vi "Facade.vi"(0 "Data In":T5 caption="数据输入", 2 "Display State In":T2 caption="显示状态输入", 3 "Container State":T4 caption="容器状态") -> (6 "Data Out":T5 caption="数据输出", 7 "Display State Out":T2 caption="显示状态输出", 8 "Action":T1 caption="动作")   [LabVIEW 2011, in "WaveFormGraph.xctl"]
uses:
  WaveFormGraph.xctl
  <vilib>/_xctls/Action.ctl
  <vilib>/_xctls/XControlSupport.lvlib
  F:/Program Files/National Instruments/LabVIEW 2011/resource/importtools/Common/Event/NISAST Event.lvclass
  <vilib>/_xctls/Container State.ctl
  Data.ctl
  State.ctl
  CursorPosQueueCluster.ctl
panel:
  out "趋势图":dbl[](graph)
  out "细节图":dbl[](graph)
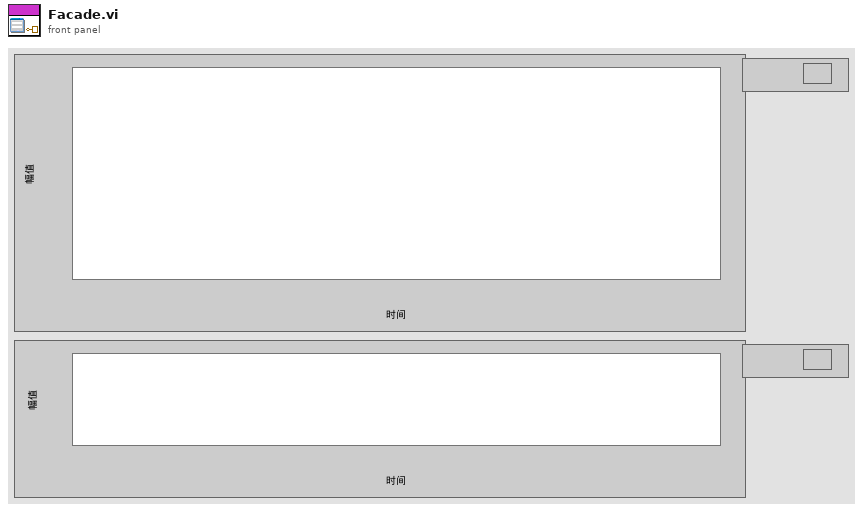
[diagram p1: front panel]
types:
  T1 = typedef "XControlSupport.lvlib/Action.ctl" = cluster{"Data Changed?":bool, "State Changed?":bool, "Action Name":string}
  T2 = typedef "WaveFormGraph.xctl/State.ctl" = cluster{"UsrEvent":refnum<class "NISAST Event.lvclass">, "游标位置":T3, "DaemRef":refnum<vi>}
  T3 = typedef "CursorPosQueueCluster.ctl" = cluster{"Cur1":refnum<queue>, "Cur2":refnum<queue>}
  T4 = typedef "XControlSupport.lvlib/Container State.ctl" = cluster{"Indicator?":bool, "Run Mode?":bool, " Refnum":refnum<vi>}
  T5 = typedef "WaveFormGraph.xctl/Data.ctl" = dbl[][]
  T6 = typedef "NISAST Event.lvclass/Event Registeration Refnum.ctl" = refnum<event-registration>
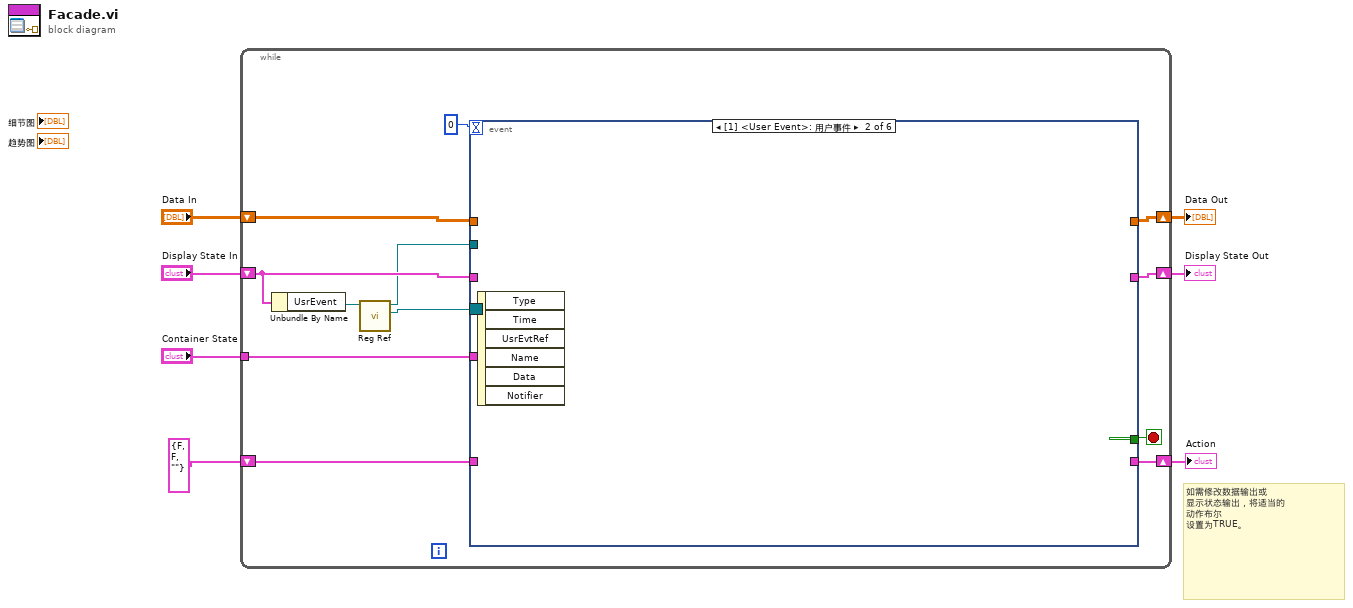
[diagram p0: block diagram]
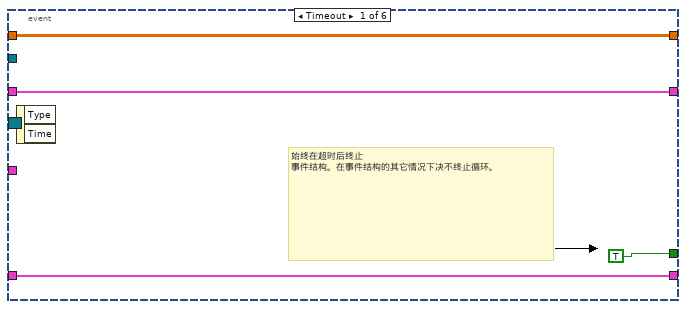
[diagram p2: hidden frame]
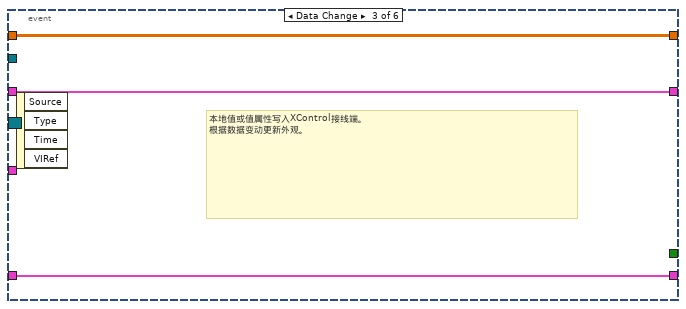
[diagram p3: hidden frame]
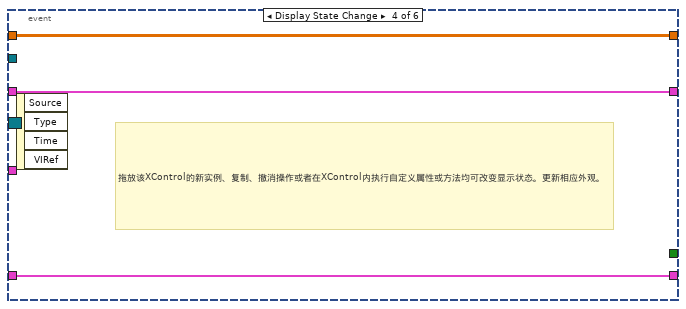
[diagram p4: hidden frame]
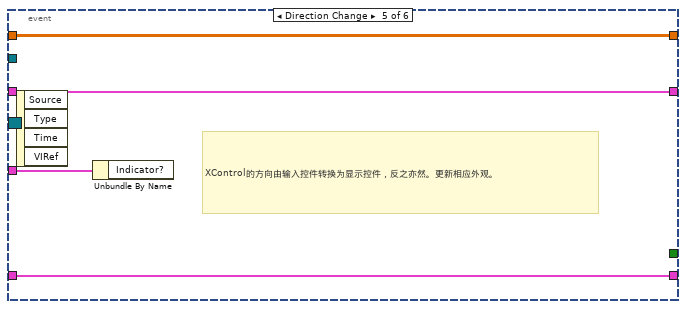
[diagram p5: hidden frame]
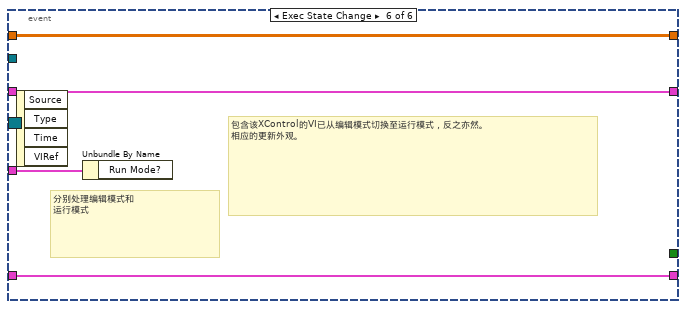
[diagram p6: hidden frame]
diagram:
  # "如需修改数据输出或\n显示状态输出，将适当的\n动作布尔\n设置为TRUE。"
  n1 = while {
    shift-right: [w19] -> w4
    shift-left: "Display State In" -> [w11]
    tunnel: "Container State" -> [w16]
    shift-right: [w14] -> w7
    shift-left: "Data In" -> [w15]
    shift-right: [w12] -> w2
    shift-left: T1 {"Data Changed?"=FALSE, "State Changed?"=FALSE, "Action Name"=""} ("Action") -> [w13]
    stop <- w18 stop-if-true
    n2 = Unbundle By Name(w11) -> ("UsrEvent"=w10:refnum<class "NISAST Event.lvclass">)
    n3 = call-dynamic "Reg Ref.vi"("Event in"=w10) -> ("Event Registration Refnum"=w9:T6, "Event out"=w8:refnum<class "NISAST Event.lvclass">)  [unwired: 8 in, 1 out]
    n4 = event shown="[1] <User Event>: 用户事件" {
      selector: w9 -> [_ _ _ _ _ _]
      dyn-events: _ -> [_ _ _ _ _ _]
      timeout: 0 -> [_ _ _ _ _ _]
      tunnel: w11 -> [w21 _ w25 w29 w32 w36]
      tunnel: [w21 _ w25 w29 w32 w36] -> w19
      tunnel: [TRUE _ _ _ _ _] -> w18
      tunnel: w16 -> [_ _ _ _ w33 w37]
      tunnel: w15 -> [w20 _ w26 w28 w31 w35]
      tunnel: [w20 _ w26 w28 w31 w35] -> w14
      tunnel: [w22 _ w24 w27 w30 w34] -> w12
      tunnel: w13 -> [w22 _ w24 w27 w30 w34]
      tunnel: w8 -> [_ _ _ _ _ _]
      event Timeout {
        # "始终在超时后终止\n事件结构。在事件结构的其它情况下决不终止循环。"
        n5 = event-data() -> ()  [unwired: 1 in, 2 out]
      }
      event User Event {
        n6 = event-data() -> ()  [unwired: 1 in, 6 out]
      }
      event Data Change {
        # "本地值或值属性写入XControl接线端。\n根据数据变动更新外观。"
        n7 = event-data() -> ()  [unwired: 1 in, 4 out]
      }
      event Display State Change {
        # "拖放该XControl的新实例、复制、撤消操作或者在XControl内执行自定义属性或方法均可改变显示状态。更新相应外观。"
        n8 = event-data() -> ()  [unwired: 1 in, 4 out]
      }
      event Direction Change {
        # "XControl的方向由输入控件转换为显示控件，反之亦然。更新相应外观。"
        n9 = event-data() -> ()  [unwired: 1 in, 4 out]
        n10 = Unbundle By Name(w33) -> ()  [unwired: 1 out]
      }
      event Exec State Change {
        # "包含该XControl的VI已从编辑模式切换至运行模式，反之亦然。\n相应的更新外观。"
        # "分别处理编辑模式和\n运行模式"
        n11 = event-data() -> ()  [unwired: 1 in, 4 out]
        n12 = Unbundle By Name(w37) -> ()  [unwired: 1 out]
      }
    }
  }
  "Display State Out" <- w4
  "Data Out" <- w7
  "Action" <- w2
